vi "Exercise1.vi"() -> ()   [LabVIEW 2019]
panel:
  out "Motor":bool
  out "Alarm":bool
  in  "Password":string
  in  "Username":string
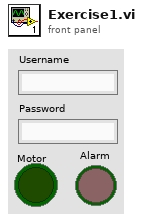
[diagram p1: front panel]
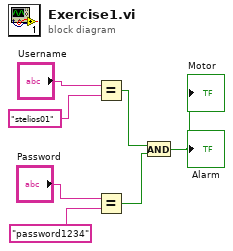
[diagram p0: block diagram]
diagram:
  n1 = Equal?(x="Username", y="stelios01") -> (x = y?=w3:bool)
  n2 = Equal?(x="Password", y="password1234") -> (x = y?=w2:bool)
  n3 = And(x=w3, y=w2) -> (x .and. y?=→"Alarm" →"Motor":bool)
